vi "TestSignal.vi"() -> ()   [LabVIEW 2011]
doc: "I. Description:\nThis example demonstrates how to acquire a finite amount of data (Waveform) using a digital reference trigger.\n\nII. Instructions for Running:\n1. Select the Physical Channel to correspond to where your signal is input on the DAQ device.\n2. Enter the Minimum and Maximum Voltage Ranges.\nNote: For better accuracy try to match the Input Ranges to the expected voltage level of the measured signal.\n3. Select how many Samples to Acquire on Each Channel. \n4. Set the Rate of the Acquisition. Note: The Rate should be AT LEAST twice as fast as the maximum frequency component of the signal being acquired.\n5. Select the Source and Edge of the Digital Reference Trigger for the acquisition.\n\nIII. Block Diagram Steps:\n1. Create an analog input voltage channel.\n2. Define the parameters for an Internal Clock Source. Additionally, define the sample mode to be Finite.\n3. Define the parameters for a Digital Edge Reference Trigger.\n4. Call the Start VI to begin the acquisition.\n5. Use the Read VI to retrieve the waveform. Set a timeout so an error is returned if the samples are not returned in the specified time limit. Note: This example reads data from one or more channels and returns an array of data. Use the Index Array function to access an individual channel of data.\n6. Call the Clear Task VI to clear the Task.\n7. Call the Trigger Cursor VI to place a vertical cursor on the graph at the x-index of the reference trigger. *Note - This VI can be removed from the block diagram without affecting the acquisition.\n8. Use the popup dialog box to display an error if any.\n\nIV. I/O Connections Overview:\nMake sure your signal input terminal matches the Physical Channel I/O Control. Also, make sure your digital trigger terminal matches the Trigger Source Control. For further connection information, refer to your hardware reference manual."
uses:
  <vilib>/Utility/error.llb/DialogType.ctl
  <vilib>/DAQmx/read.llb/DAQmx Read (Analog 1D Wfm NChan NSamp).vi
  <vilib>/DAQmx/create/channels.llb/DAQmx Create Channel (AI-Voltage-Basic).vi
  <vilib>/DAQmx/configure/timing.llb/DAQmx Timing (Sample Clock).vi
  <vilib>/DAQmx/configure/trigger.llb/DAQmx Reference Trigger (Digital Edge).vi
  <vilib>/DAQmx/miscellaneous.llb/DAQmx Fill In Error Info.vi
panel:
  in  "Trigger Source":tag="/Dev1/Ctr0InternalOutput"
  in  "Maximum Value":dbl=10.0 format="%0.2f"
  in  "Minimum Value":dbl=-10.0 format="%0.2f"
  in  "Physical Channel":tag="Dev1/ai1:3"
  out "Measurement":waveform(dbl)[](graph)=[{"t0"=timestamp(3493191884.3729534 s since 1904-01-01), "dt"=9.999999999999999e-05, "Y"=array[25000 elements], "attributes"=variant("NI_ChannelName"=variant(string "Dev1/ai1"), "NI_UnitDescription"=variant(string "Volts"))}, {"t0"=timestamp(3493191884.3729644 s since 1904-01-01), "dt"=9.999999999999999e-05, "Y"=array[25000 elements], "attributes"=variant("NI_ChannelName"=variant(string "Dev1/ai2"), "NI_UnitDescription"=variant(string "Volts"))}, {"t0"=timestamp(3493191884.3729753 s since 1904-01-01), "dt"=9.999999999999999e-05, "Y"=array[25000 elements], "attributes"=variant("NI_ChannelName"=variant(string "Dev1/ai3"), "NI_UnitDescription"=variant(string "Volts"))}]
  # "For instructions, select Help>>Show Context Help"
  # "Channel Parameters"
  # "Ctr0 for Red trigger\nCtr1 for Green trigger"
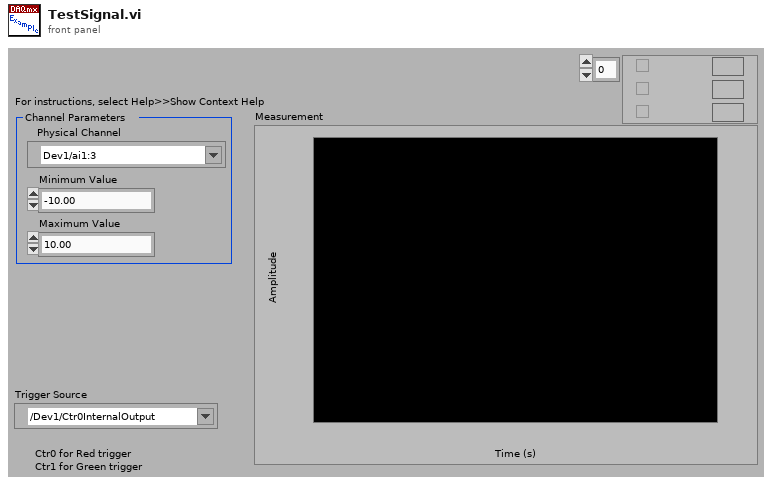
[diagram p1: front panel]
types:
  T1 = typedef "DialogType.ctl" = u16
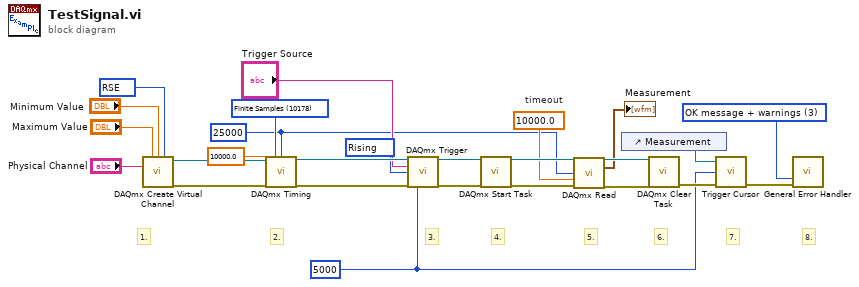
[diagram p0: block diagram]
diagram:
  w8 = 25000 ("Samples per Channel")
  w5 = u32 5000 ("Pre-Trigger Samples")
  w12 = 10280 items=["Rising"=10280, "Falling"=10171] ("Edge")
  w1 = 10083 items=["default"=-1, "RSE"=10083, "NRSE"=10078, "Differential"=10106, "Pseudodifferential"=12529] ("input terminal configuration")
  w2 = T1 3 items=["no dialog", "OK message", "continue or stop message", "OK message + warnings", "continue/stop + warnings"] ("type of dialog (OK msg:1)")
  w10 = 10000.0  # timeout
  w11 = 10178 items=["Finite Samples"=10178, "Continuous Samples"=10123] ("sample mode")
  # "8."
  # "7."
  # "5."
  # "6."
  # "4."
  # "3."
  # "2."
  # "1."
  n1 = call-poly <vilib>:"DAQmx Create Virtual Channel.vi"("maximum value"="Maximum Value", "minimum value"="Minimum Value", "input terminal configuration"=w1, "physical channels"="Physical Channel") -> ("task out"=w18:refnum<k21>, "error out"=w24:errorcluster)  [unwired: 5 in, 5 out]
  n2 = call-poly <vilib>:"DAQmx Timing.vi"("task/channels in"=w18, "sample mode"=w11, "samples per channel"=w8, "rate"=10000.0 ("Rate"), "error in"=w24) -> ("task out"=w17:refnum<k21>, "error out"=w23:errorcluster)  [unwired: 2 in, 7 out]
  n3 = call-poly <vilib>:"DAQmx Trigger.vi"("task/channels in"=w17, "source"="Trigger Source", "edge"=w12, "error in"=w23, "pretrigger samples per channel"=w5) -> ("task out"=w16:refnum<k21>, "error out"=w22:errorcluster)  [unwired: 9 out]
  n4 = call <vilib>:"DAQmx Start Task.vi"("task/channels in"=w16, "error in"=w22) -> ("task out"=w15:refnum<k21>, "error out"=w21:errorcluster)  [unwired: 12 out]
  n5 = call-poly <vilib>:"DAQmx Read.vi"("task/channels in"=w15, "number of samples per channel"=w8, "timeout"=w10, "error in"=w21) -> ("task out"=w14:refnum<k21>, "data"=→"Measurement":waveform(dbl)[], "error out"=w20:errorcluster)  [unwired: 9 out]
  n6 = control-ref of="Measurement"() -> (w3:refnum<vi>)
  n7 = call <vilib>:"DAQmx Clear Task.vi"("task in"=w14, "error in"=w20) -> ("error out"=w7:errorcluster)  [unwired: 13 out]
  n8 = call "Trigger Cursor.vi"("error in (no error)"=w7, "Pre-Trigger Scans"=w5, "Waveform Graph Reference"=w3) -> ("error out"=w6:errorcluster)
  n9 = call <vilib>:"General Error Handler.vi"("type of dialog (OK msg:1)"=w2, "error in (no error)"=w6) -> ()  [unwired: 14 out]
